vi "prueba_serie_labview1.vi"() -> ()   [LabVIEW 2015]
uses:
  <vilib>/Instr/_visa.llb/VISA Configure Serial Port (Instr).vi
panel:
  in  "Menus":enum32{"Configuración", "Variables", "Graficas"}(tab)
  in  "LECTURA":bool
  in  "ESCRITURA":bool
  in  "Stop Button 2":bool
  in  "VISA resource name":refnum<visa-resource-name>
  out "read buffer":string
  in  "number":dbl
  out "Numeric":dbl
  in  "ms":dbl=0.1
  out "Al PIC":string
  out "Array":dbl[](array[numeric])
  out "Waveform Chart":dbl(graph)
  # "ELECTROCARDIOGRAFO \nPORTATIL"
  # "(Seg)"
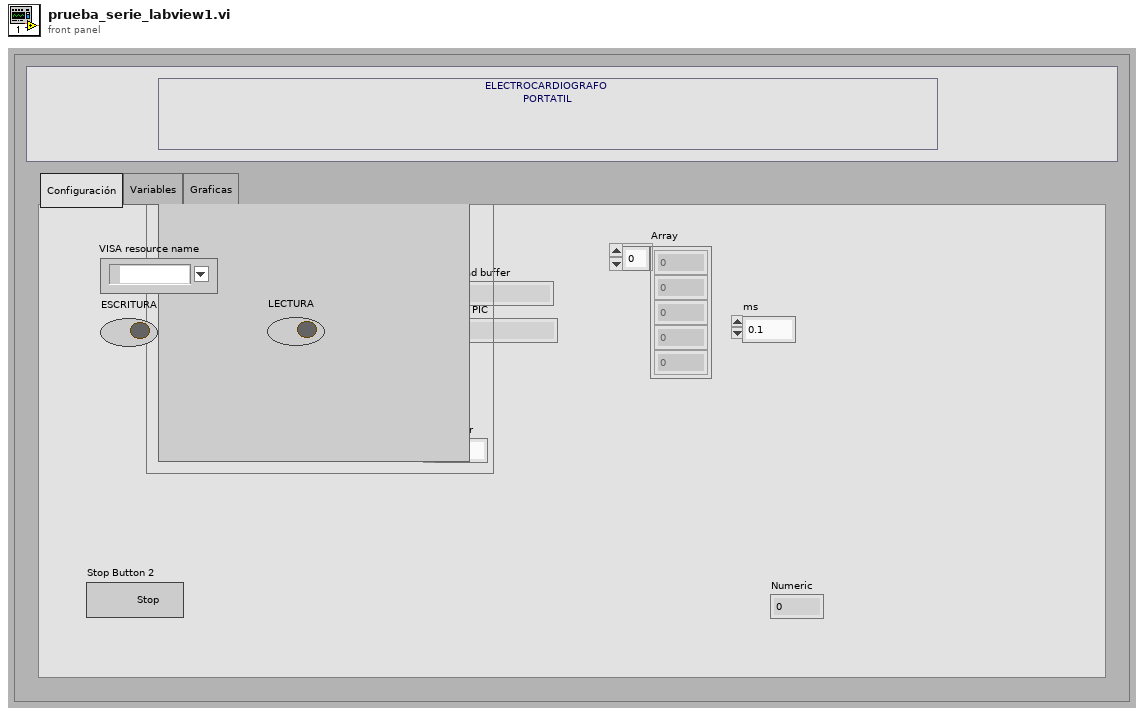
[diagram p1: front panel]
types:
  T1 = cluster{"unsigned byte array[0]":u8, "unsigned byte array[1]":u8, "unsigned byte array[2]":u8, "unsigned byte array[3]":u8, "unsigned byte array[4]":u8, "unsigned byte array[5]":u8, "unsigned byte array[6]":u8, "unsigned byte array[7]":u8, "unsigned byte array[8]":u8}
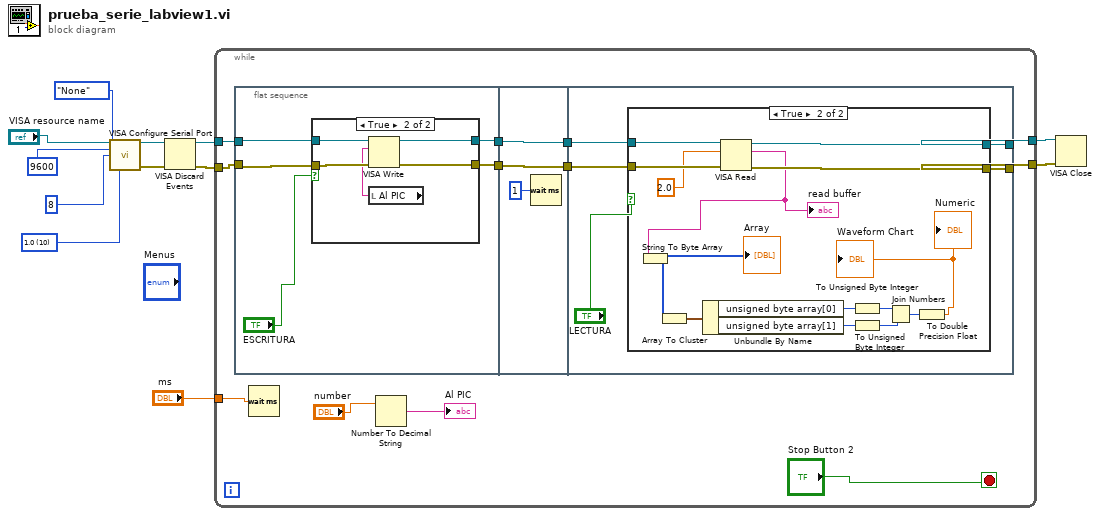
[diagram p0: block diagram]
diagram:
  w8 = u16 10 items=["1.0"=10, "1.5"=15, "2.0"=20] ("stop bits (10: 1 bit)")
  n1 = call-poly "VISA Configure Serial Port"("VISA resource name"="VISA resource name", "baud rate (9600)"=9600 ("Numeric 2"), "data bits (8)"=u16 8, "parity (0:none)"=enum16{"None", "Odd", "Even", "Mark", "Space"}."None", "stop bits (10: 1 bit)"=w8) -> ("VISA resource name out"=w7:refnum<visa-resource-name>, "error out"=w6:errorcluster)  [unwired: 9 in]
  n2 = VISA Discard Events(8:w6, 11:w7) -> (0:w4:errorcluster, 3:w5:refnum<visa-resource-name>)  [unwired: 2 in]
  n3 = while {
    tunnel: w5 -> [w20]
    tunnel: [w19] -> w11
    tunnel: [w18] -> w10
    tunnel: w4 -> [w15]
    tunnel: "ms" -> [w13]
    stop <- "Stop Button 2" stop-if-true
    n4 = flat-sequence {
      tunnel: w20 -> [w29]
      tunnel: [w28] -> w24
      tunnel: [w27] -> w23
      tunnel: w15 -> [w26]
      tunnel: [w39] -> w22
      tunnel: w24 -> [w39]
      tunnel: w23 -> [w38]
      tunnel: [w38] -> w21
      tunnel: w22 -> [w44]
      tunnel: [w43] -> w19
      tunnel: [w42] -> w18
      tunnel: w21 -> [w41]
      frame #0 {
        n5 = case shown="True" "ESCRITURA" {
          tunnel: w29 -> [w31 w36]
          tunnel: [w31 w32] -> w28
          tunnel: [w30 w35] -> w27
          tunnel: w26 -> [w30 w34]
          frame False {
          }
          frame True {
            n6 = local read "Al PIC"() -> (w33:string)
            n7 = VISA Write(VISA resource name=w36, write buffer=w33, error in (no error)=w34) -> (VISA resource name out=w32:refnum<visa-resource-name>, error out=w35:errorcluster)  [unwired: 1 out]
          }
        }
      }
      frame #1 {
        n8 = Wait (ms)(milliseconds to wait=u32 1) -> ()  [unwired: 1 out]
      }
      frame #2 {
        n9 = case shown="True" "LECTURA" {
          tunnel: w44 -> [w46 w60]
          tunnel: [w46 w59] -> w43
          tunnel: [w45 w58] -> w42
          tunnel: w41 -> [w45 w57]
          frame False {
          }
          frame True {
            n10 = VISA Read(VISA resource name=w60, byte count=2.0 ("BYTES A LEER"), error in (no error)=w57) -> (VISA resource name out=w59:refnum<visa-resource-name>, read buffer=w56:string, error out=w58:errorcluster)  [unwired: 1 out]
            "read buffer" <- w56
            n11 = String To Byte Array(string=w56) -> (unsigned byte array=w55:u8[])
            "Array" <- w55
            n12 = Array To Cluster(array=w55) -> (cluster=w54:T1)
            n13 = Unbundle By Name(w54) -> ("unsigned byte array[0]"=w50:u8, "unsigned byte array[1]"=w49:u8)
            n14 = To Unsigned Byte Integer(number=w50) -> (unsigned 8bit integer=w53:u8)
            n15 = To Unsigned Byte Integer(number=w49) -> (unsigned 8bit integer=w52:u8)
            n16 = Join Numbers(hi=w53, lo=w52) -> ((hi.lo)=w51:u16)
            n17 = To Double Precision Float(number=w51) -> (double precision float=→"Numeric" →"Waveform Chart":dbl)
          }
        }
      }
    }
    n18 = Wait (ms)(milliseconds to wait=w13) -> ()  [unwired: 1 out]
    n19 = Number To Decimal String(number="number") -> (decimal integer string=→"Al PIC":string)  [unwired: 1 in]
  }
  n20 = VISA Close(VISA resource name=w11, error in (no error)=w10) -> ()  [unwired: 1 out]
